vi "Is Optimized.vi"(8 "Error In":errorcluster, 11 "Tree Manager":refnum<data-value>) -> (0 "Error Out":errorcluster, 1 "Is Optimized?":bool, 3 "Tree Manager":refnum<data-value>)   [LabVIEW 2017, in "Tree API.lvlib" / "Tree.lvclass"]
doc: "Check if the Tree is optimized for searching. If it is not you can call the Optimize Search method. Every modification of the Tree structure resets this flag.s"
uses:
  Tree.lvclass
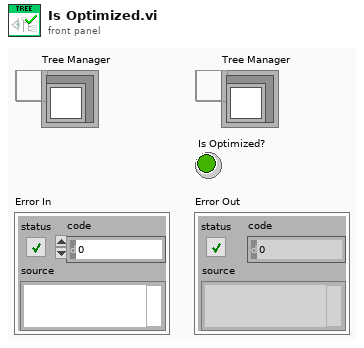
[diagram p1: front panel]
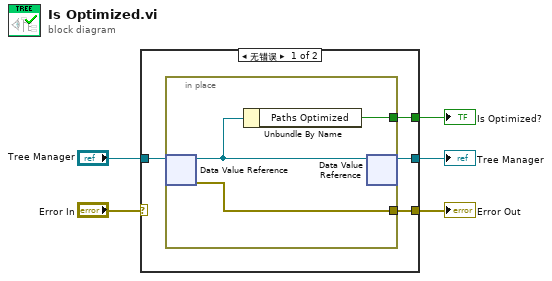
[diagram p0: block diagram]
diagram:
  n1 = case shown="无错误" "Error In" {
    selector: "Error In" -> [_ w13]
    tunnel: "Tree Manager" -> [w9 w14]
    tunnel: [w8 w14] -> w4
    tunnel: [w7 w13] -> w2
    tunnel: [w6 _] -> w1
    frame No Error {
      n2 = in-place {
        in-place-border: [w12] -> w7
        in-place-border: [w10] -> w6
        n3 = in-place-dvr #1(w9) -> (w11:refnum<class "Tree.lvclass">, w12:errorcluster)
        n4 = Unbundle By Name(w11) -> ("Paths Optimized"=w10:bool)
        n5 = in-place-dvr #1(w11) -> (w8:refnum<data-value>)  [unwired: 1 out]
      }
    }
    frame Error {
    }
  }
  "Tree Manager" <- w4
  "Error Out" <- w2
  "Is Optimized?" <- w1
